vi "auto_ctrl_run_valve_with_flow.vi"(6 "ref_sp_turn":refnum<vi>, 7 "array_value_in":dbl[](array[numeric]) format="%.2f", 9 "flow_set":dbl=3.0 format="%.1f", 10 "enable_auto_ctrl":bool caption="Auto Control") -> (0 "turn_new":dbl format="%.3f", 1 "status":u32(colorbox), 5 "array_value_out":dbl[](array[numeric]))   [LabVIEW 2019]
doc: "This example demonstrates how to simulate a general PID controller."
uses:
  <vilib>/Analysis/baseanly.llb/Mean (DBL).vi
  THCD_401/THCD_401_Global.vi
  <vilib>/addons/control/pid/pid.llb/PID (DBL).vi
  <vilib>/addons/control/pid/NI_PID_pid.lvlib
  <vilib>/Analysis/NI_AALBase.lvlib
panel:
  out "level_used":dbl format="%0.2f"
  in  "n_avg":u8=30
  in  "control_step":dbl=0.01 format="%#_13g"
  in  "turn_nominal":dbl=1.0 format="%.2f"
  in  "turn_max":dbl=2.0 format="%.2f"
  in  "turn_min":dbl=0.3 format="%.2f"
  out "MV":dbl format="%.1f"
  out "PID Range":cluster{"High":dbl, "Low":dbl} {"Low" format="%.1f"; "High" format="%.1f"}
  in  "PID gains":T1={"proportional gain (Kc)"=0.1, "integral time (Ti, min)"=1.0, "derivative time (Td, min)"=0.5} {"derivative time (Td, min)" format="%.4f"; "integral time (Ti, min)" format="%.4f"; "proportional gain (Kc)" format="%.3f"}
  # "Kc = delta_turn / delta_flow ~ 0.1 / 1.0 = 0.1\nTi: 0.5 -> 1.0\nTd: 0.2 -> 0.5"
  # "turn"
  # "turn"
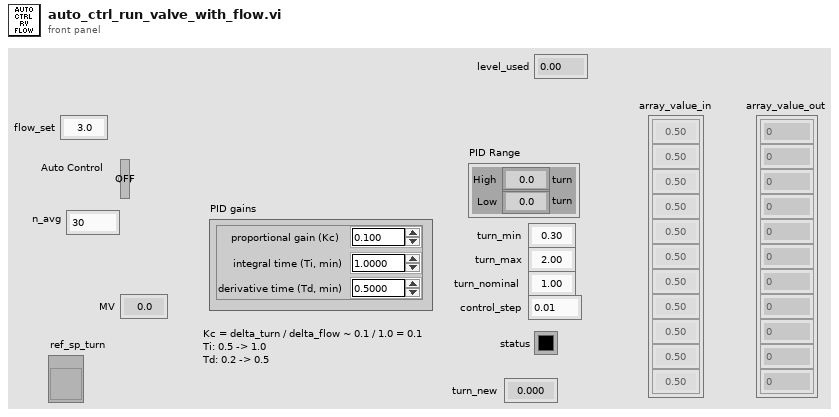
[diagram p1: front panel]
types:
  T1 = cluster{"proportional gain (Kc)":dbl, "integral time (Ti, min)":dbl, "derivative time (Td, min)":dbl}
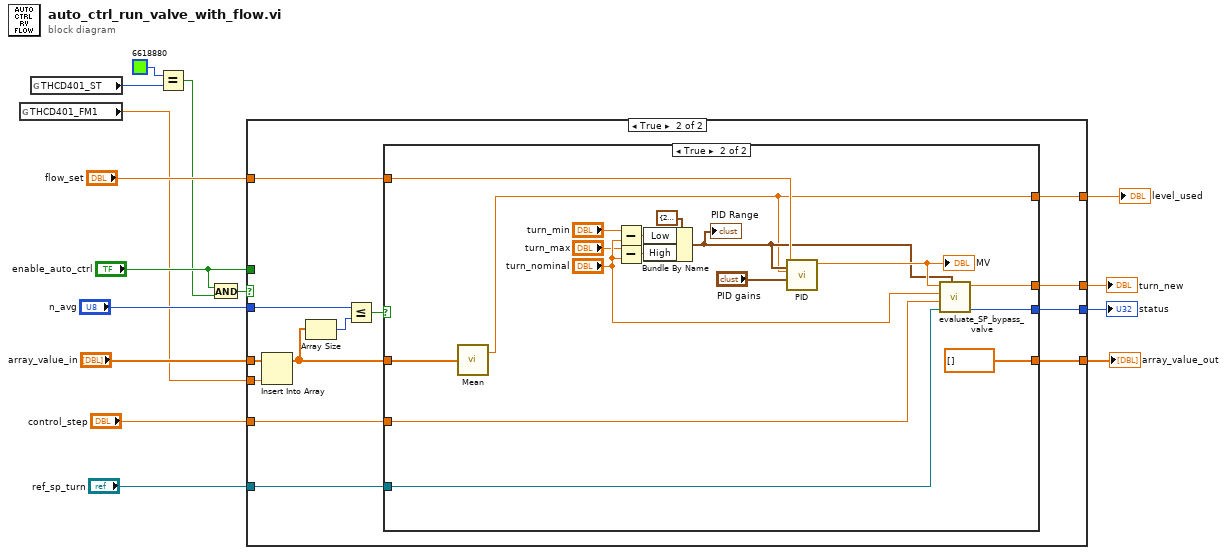
[diagram p0: block diagram]
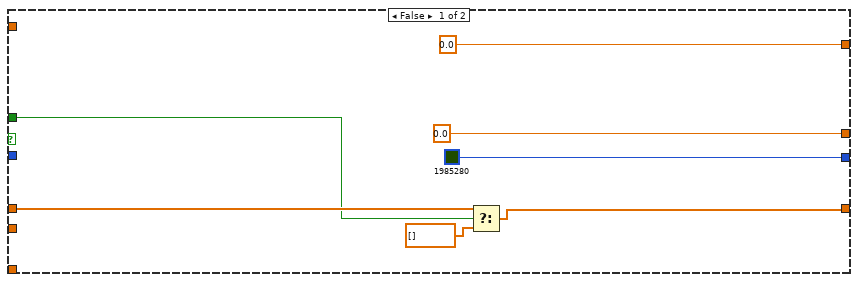
[diagram p2: hidden frame]
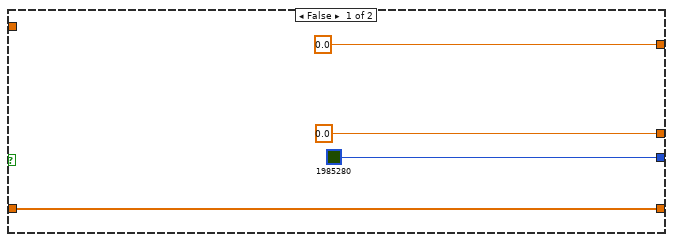
[diagram p3: hidden frame]
diagram:
  n1 = global read "THCD_401_Global.vi" "THCD401_FM1"() -> (w1:dbl)
  n2 = global read "THCD_401_Global.vi" "THCD401_ST"() -> (w5:u32)
  n3 = Equal?(x=u32 6618880 ("THCD401_ST"), y=w5) -> (x = y?=w4:bool)
  n4 = And(x="enable_auto_ctrl", y=w4) -> (x .and. y?=w11:bool)
  n5 = case shown="True" w11 {
    tunnel: [0.0 ("F_O_new") w33] -> w15
    tunnel: [u32 1985280 ("alarm_status") w35] -> w14
    tunnel: "flow_set" -> [_ w32]
    tunnel: "ref_sp_turn" -> [_ w34]
    tunnel: "control_step" -> [_ w31]
    tunnel: [w18 w30] -> w9
    tunnel: "array_value_in" -> [w19 w25]
    tunnel: [0.0 ("mean") w29] -> w8
    tunnel: "enable_auto_ctrl" -> [w16 _]
    tunnel: "n_avg" -> [_ w27]
    tunnel: w1 -> [_ w24]
    frame False {
      n6 = Select(t=w19, s=w16, f=dbl[] []) -> (s? t:f=w18:dbl[])
    }
    frame True {
      n7 = Insert Into Array(array=w25, new element=w24) -> (w23:dbl[])  [unwired: 1 in]
      n8 = Array Size(array=w23) -> (size(s)=w28:i32)
      n9 = Less Or Equal?(x=w27, y=w28) -> (x <= y?=w26:bool)
      n10 = case shown="True" w26 {
        tunnel: [u32 1985280 ("alarm_status") w56] -> w35
        tunnel: w34 -> [_ w55]
        tunnel: [0.0 ("F_O_new") w54] -> w33
        tunnel: w32 -> [_ w52]
        tunnel: w31 -> [_ w43]
        tunnel: w23 -> [w39 w42]
        tunnel: [w39 dbl[] [] ("array_value_in")] -> w30
        tunnel: [0.0 ("mean") w40] -> w29
        frame False {
        }
        frame True {
          n11 = call-poly <vilib>:"Mean.vi"("X"=w42) -> ("mean"=w40:dbl)  [unwired: 1 out]
          n12 = Subtract(x="turn_min", y="turn_nominal") -> (x-y=w48:dbl)
          n13 = Subtract(x="turn_max", y="turn_nominal") -> (x-y=w49:dbl)
          n14 = Bundle By Name(cluster=cluster{"High":dbl, "Low":dbl} {"High"=20.0, "Low"=-20.0} ("PID Range"), "Low"=w48, "High"=w49) -> (w44:cluster{"High":dbl, "Low":dbl})
          "PID Range" <- w44
          n15 = call-poly <vilib>:"PID.vi"("output range"=w44, "PID gains"="PID gains", "process variable"=w40, "setpoint"=w52) -> ("output"=w51:dbl)  [unwired: 6 in, 1 out]
          "MV" <- w51
          n16 = call "evaluate_SP_bypass_valve.vi"("PID Range"=w44, "ref_sp_ch1"=w55, "control_step"=w43, "F_org"="turn_nominal", "control"=w51) -> ("status"=w56:u32, "F_new"=w54:dbl)  [unwired: 5 in]
        }
      }
    }
  }
  "turn_new" <- w15
  "status" <- w14
  "array_value_out" <- w9
  "level_used" <- w8
